vi "Drive for Time.vi"(0 "Startup":bool, 1 "Time to Run (ms)":dbl, 2 "Step":i32, 3 "Drive (Throttle)":dbl, 4 "Translation (Throttle)":dbl) -> (11 "Completed":bool, 12 "Back Left Spin Power":dbl, 13 "Front Right Motor Power":dbl, 14 "Back Right Spin Power":dbl, 15 "Front Left Spin Power":dbl, 16 "Front Right Spin Power":dbl, 17 "Back Left Motor Power":dbl, 18 "Back Right Motor Power":dbl, 19 "Front Left Motor Power":dbl)   [LabVIEW 2016]
uses:
  Command Execution State.ctl
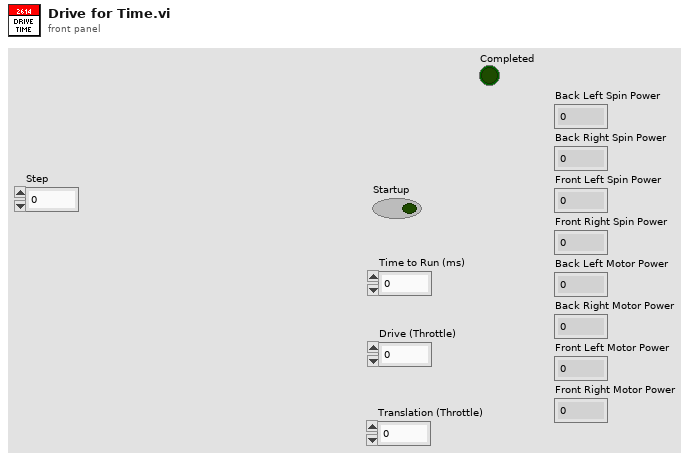
[diagram p1: front panel]
types:
  T1 = typedef "Command Execution State.ctl" = enum16{"Initialize", "Execute", "Finish"}
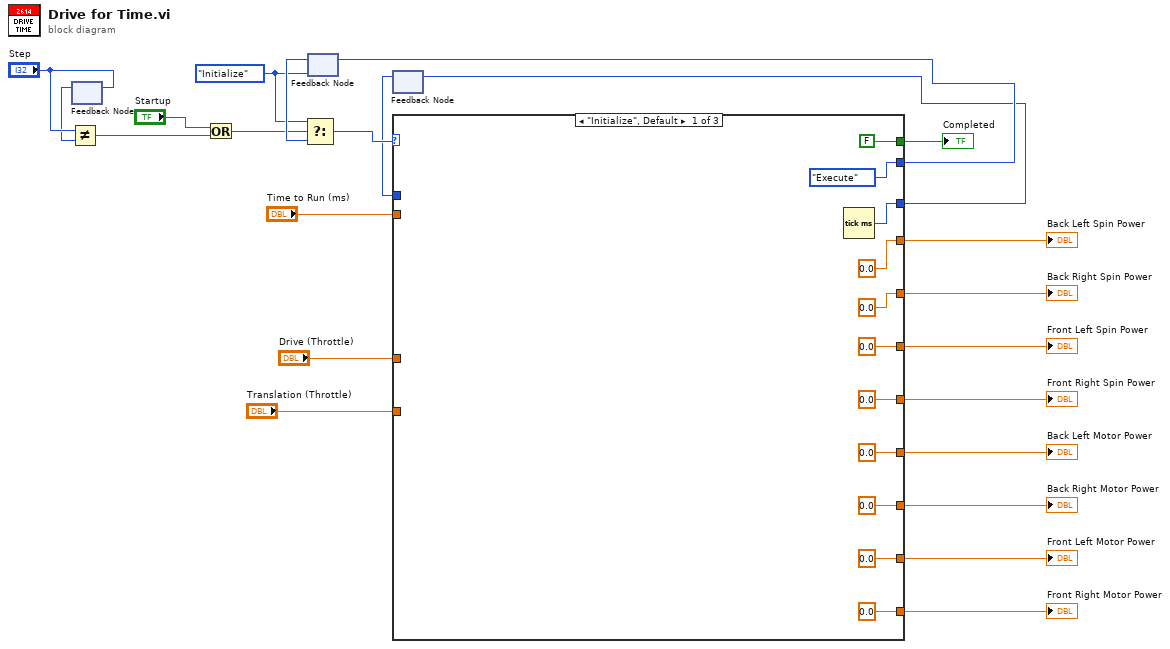
[diagram p0: block diagram]
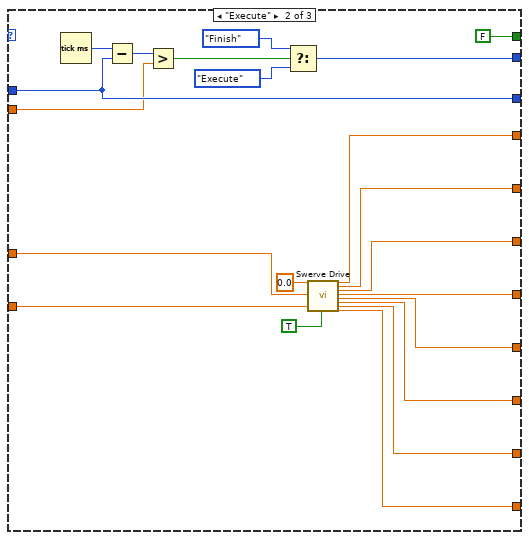
[diagram p2: hidden frame]
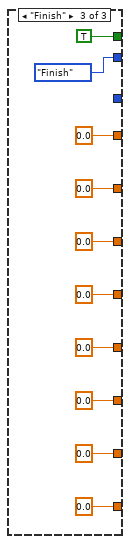
[diagram p3: hidden frame]
diagram:
  w6 = Command_Execution_State."Initialize" ("Play State")
  n1 = feedback #1() -> (w3:i32)  [unwired: 1 in]
  n2 = Not Equal?(x="Step", y=w3) -> (x != y?=w1:bool)
  n3 = feedback-in #1("Step") -> ()
  n4 = Or(x="Startup", y=w1) -> (x .or. y?=w2:bool)
  n5 = feedback #2(w6) -> (w20:T1)
  n6 = Select(t=w6, s=w2, f=w20) -> (s? t:f=w23:T1)
  n7 = feedback #3() -> (w15:u32)  [unwired: 1 in]
  n8 = case shown="\"Initialize\", Default" w23 {
    tunnel: [Command_Execution_State."Execute" ("Play State") w55 Command_Execution_State."Finish" ("Play State")] -> w21
    tunnel: "Time to Run (ms)" -> [_ w51 _]
    tunnel: "Drive (Throttle)" -> [_ w47 _]
    tunnel: "Translation (Throttle)" -> [_ w46 _]
    tunnel: [w34 w53 _] -> w16
    tunnel: w15 -> [_ w53 _]
    tunnel: [0.0 ("Back Left Spin Power") w45 0.0 ("Back Left Spin Power")] -> w14
    tunnel: [0.0 ("Back Right Spin Power") w44 0.0 ("Back Right Spin Power")] -> w13
    tunnel: [0.0 ("Front Left Spin Power") w43 0.0 ("Front Left Spin Power")] -> w12
    tunnel: [0.0 ("Front Right Spin Power") w42 0.0 ("Front Right Spin Power")] -> w11
    tunnel: [0.0 ("Back Left Motor Power") w41 0.0 ("Back Left Motor Power")] -> w7
    tunnel: [0.0 ("Back Right Motor Power") w40 0.0 ("Back Right Motor Power")] -> w8
    tunnel: [0.0 ("Front Left Motor Power") w39 0.0 ("Front Left Motor Power")] -> w9
    tunnel: [0.0 ("Front Right Motor Power") w38 0.0 ("Front Right Motor Power")] -> w10
    tunnel: [FALSE FALSE TRUE] -> w5
    frame "Initialize", Default {
      n9 = Tick Count (ms)() -> (millisecond timer value=w34:u32)
    }
    frame "Execute" {
      n10 = Tick Count (ms)() -> (millisecond timer value=w54:u32)
      n11 = Subtract(x=w54, y=w53) -> (x-y=w52:u32)
      n12 = Greater?(x=w52, y=w51) -> (0:w50:bool)
      n13 = Select(t=Command_Execution_State."Finish" ("Play State"), s=w50, f=Command_Execution_State."Execute" ("Play State")) -> (s? t:f=w55:T1)
      n14 = call "Swerve Drive.vi"("X"=0.0 ("Y"), "Y"=w47, "Z"=w46, "Robot-Centric"=TRUE) -> ("Back Left Spin Power"=w45:dbl, "Back Right Spin Power"=w44:dbl, "Front Left Spin Power"=w43:dbl, "Front Right Spin Power"=w42:dbl, "Back Left Motor Power"=w41:dbl, "Back Right Motor Power"=w40:dbl, "Front Left Motor Power"=w39:dbl, "Front Right Motor Power"=w38:dbl)  [unwired: 16 in]
    }
    frame "Finish" {
    }
  }
  "Back Left Spin Power" <- w14
  "Back Right Spin Power" <- w13
  "Front Left Spin Power" <- w12
  "Front Right Spin Power" <- w11
  "Back Left Motor Power" <- w7
  "Back Right Motor Power" <- w8
  "Front Left Motor Power" <- w9
  "Front Right Motor Power" <- w10
  "Completed" <- w5
  n15 = feedback-in #2(w21) -> ()
  n16 = feedback-in #3(w16) -> ()
